vi "FL_Save_incrementally.vi"(0 "Temporary file output path":path, 1 "Record / Stop record":bool, 2 "Exit acquisition loop":bool, 5 "Loop iteration":i32, 7 "Loop speed in ms":u16, 9 "Save every N seconds":u32=15, 11 "error in (no error)":errorcluster, 12 "Sensor read input":T1(array[cluster])) -> (4 "Eff. save interval":sgl, 15 "error out":errorcluster)   [LabVIEW 2016]
panel:
  in  "Max chunk size":i64=50331648
  in  "Number of the file chunk":i32
  out "Chunk size (in bytes)":i64
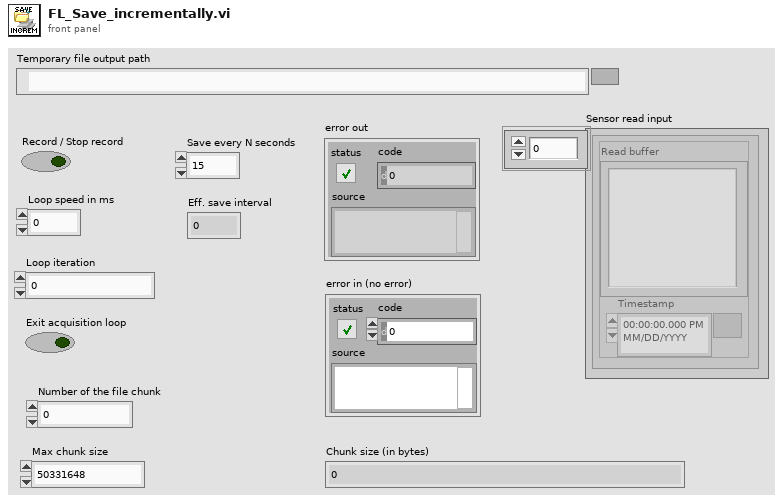
[diagram p1: front panel]
types:
  T1 = cluster{"Read buffer":string, "Timestamp":timestamp}[]
  T2 = enum16{"open", "replace", "create", "open or create", "replace or create", "replace or create with confirmation"}
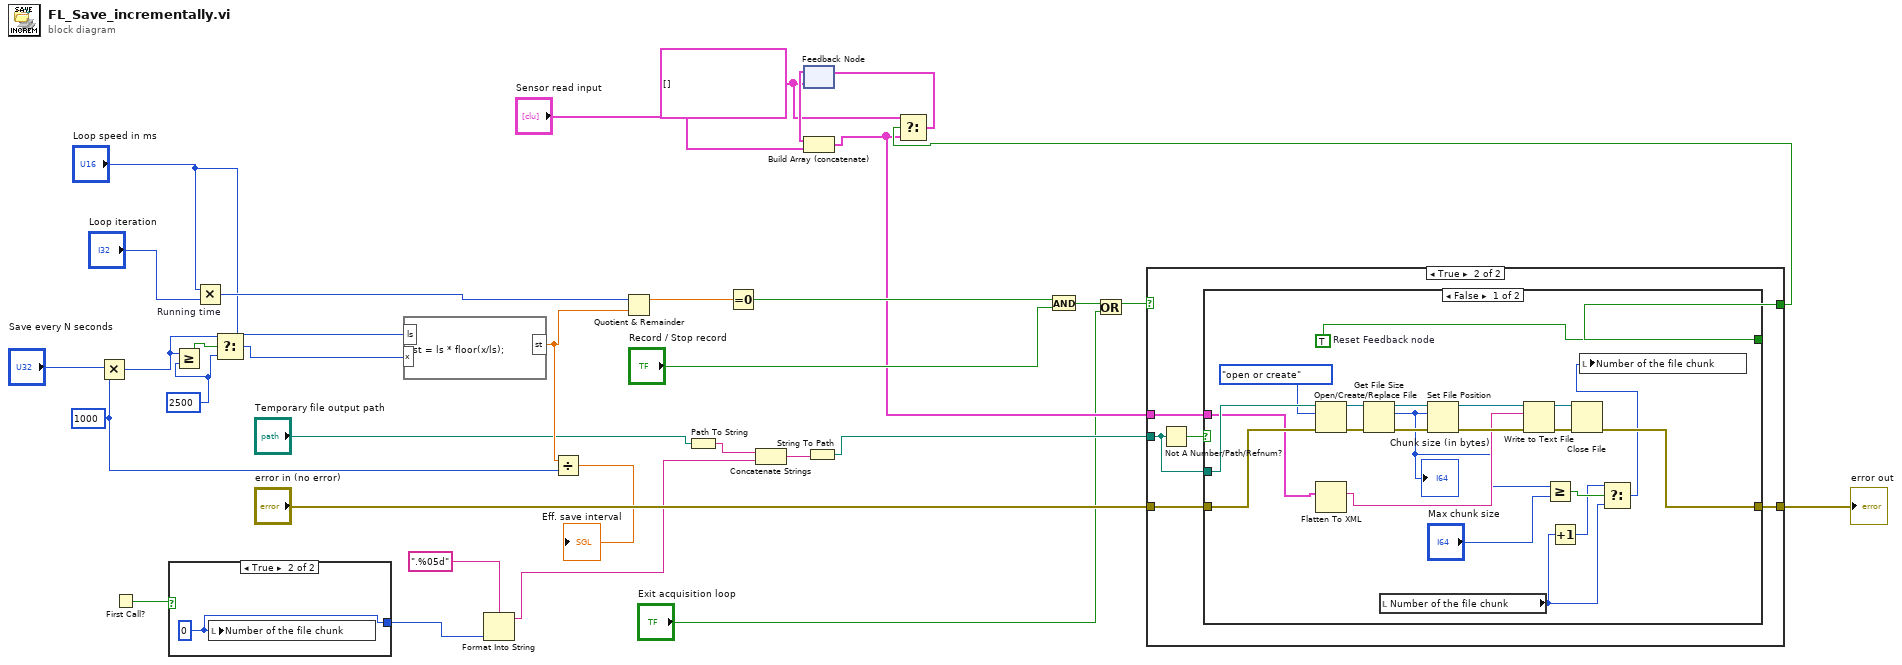
[diagram p0: block diagram]
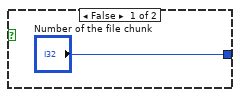
[diagram p2: hidden frame]
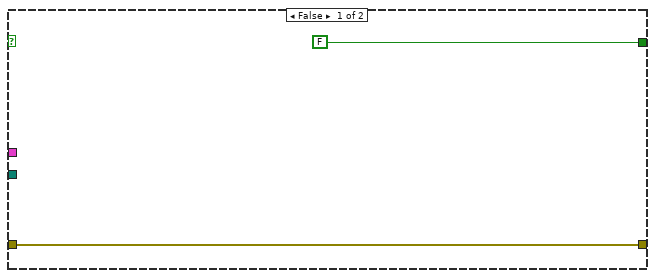
[diagram p3: hidden frame]
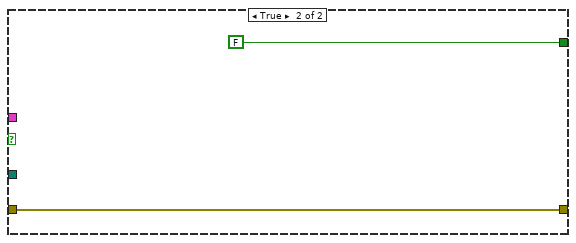
[diagram p4: hidden frame]
diagram:
  w12 = T1 []
  w17 = u32 1000 ("y")
  w24 = 2500
  n1 = Multiply(x="Save every N seconds", y=w17) -> (x*y=w20:u32)
  n2 = First Call?() -> (First Call?: T/F=w3:bool)
  n3 = case shown="True" w3 {
    tunnel: ["Number of the file chunk" w35] -> w2
    frame False {
    }
    frame True {
      w35 = 0 ("Number of the file chunk")
      n4 = local write "Number of the file chunk"(w35) -> ()
    }
  }
  n5 = Greater Or Equal?(x=w20, y=w24) -> (x >= y?=w25:bool)
  n6 = Multiply "Running time"(x="Loop speed in ms", y="Loop iteration") -> (x*y=w30:i32)
  n7 = Select(t=w20, s=w25, f=w24) -> (s? t:f=w22:u32)
  n8 = formula code="st = ls * floor(x/ls);"("ls"="Loop speed in ms", "x"=w22) -> ("st"=w19:dbl)
  n9 = Format Into String(format string=".%05d", w2) -> (resulting string=w6:string)  [unwired: 2 in, 1 out]
  n10 = Divide(x=w19, y=w17) -> (x/y=→"Eff. save interval":dbl)
  n11 = Quotient & Remainder(x=w30, y=w19) -> (x-y*floor(x/y)=w28:dbl)  [unwired: 1 out]
  n12 = Path To String(path="Temporary file output path") -> (string=w7:string)
  n13 = Equal To 0?(x=w28) -> (x = 0?=w29:bool)
  n14 = Concatenate Strings(w7, w6) -> (w5:string)
  n15 = feedback #1(w12) -> (w14:T1)
  n16 = Build Array (concatenate)(w14, "Sensor read input") -> (w10:T1)
  n17 = String To Path(string=w5) -> (path=w4:path)
  n18 = And(x=w29, y="Record / Stop record") -> (x .and. y?=w33:bool)
  n19 = Or(x=w33, y="Exit acquisition loop") -> (x .or. y?=w16:bool)
  n20 = case shown="True" w16 {
    tunnel: w4 -> [_ w42]
    tunnel: [FALSE w41] -> w11
    tunnel: "error in (no error)" -> [w36 w40]
    tunnel: [w36 w39] -> w26
    tunnel: w10 -> [_ w38]
    frame False {
    }
    frame True {
      n21 = Not A Number/Path/Refnum?(number/path/refnum=w42) -> (NaN/Path/Refnum?=w43:bool)
      n22 = case shown="False" w43 {
        tunnel: w42 -> [w57 _]
        tunnel: [w64 FALSE] -> w41
        tunnel: w40 -> [w52 w65]
        tunnel: [w53 w65] -> w39
        tunnel: w38 -> [w51 _]
        frame False {
          w64 = TRUE  # Reset Feedback node
          n23 = Open/Create/Replace File(file path (use dialog)=w57, error in=w52, operation (0:open)=T2."open or create") -> (refnum out=w58:refnum<file>, error out=w59:errorcluster)  [unwired: 3 in, 1 out]
          n24 = Flatten To XML(anything=w51) -> (xml string=w50:string)
          n25 = Get File Size(file=w58, error in=w59) -> (refnum out=w62:refnum<file>, size (in bytes)=w49:i64, 0:w63:errorcluster)
          "Chunk size (in bytes)" <- w49
          n26 = local read "Number of the file chunk"() -> (w45:i32)
          n27 = Set File Position(offset (in bytes) (0)=w49, refnum=w62, error in=w63) -> (refnum out=w60:refnum<file>, error out=w61:errorcluster)  [unwired: 1 in]
          n28 = Write to Text File(file (use dialog)=w60, text=w50, error in=w61) -> (refnum out=w54:refnum<file>, error out=w55:errorcluster)  [unwired: 1 in, 1 out]
          n29 = Greater Or Equal?(x=w49, y="Max chunk size") -> (x >= y?=w47:bool)
          n30 = Increment(x=w45) -> (x+1=w46:i32)
          n31 = Close File(refnum=w54, error in=w55) -> (error out=w53:errorcluster)  [unwired: 1 out]
          n32 = Select(t=w46, s=w47, f=w45) -> (s? t:f=w44:i32)
          n33 = local write "Number of the file chunk"(w44) -> ()
        }
        frame True {
        }
      }
    }
  }
  "error out" <- w26
  n34 = Select(t=w12, s=w11, f=w10) -> (s? t:f=w13:T1)
  n35 = feedback-in #1(w13) -> ()
